vi "MakeMatlabParameterBundle.vi"(9 "value":variant, 10 "name":string, 11 "MatlabType":T2) -> (3 "MatlabDataBundle":T1)   [LabVIEW 2017]
uses:
  Types/MatlabDataType.ctl
  Types/MatlabDataBundle.ctl
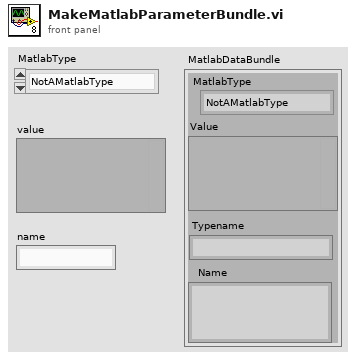
[diagram p1: front panel]
types:
  T1 = typedef "MatlabDataBundle.ctl" = cluster{"MatlabType":T2, "Value":variant, "Name":string, "Typename":string}
  T2 = typedef "MatlabDataType.ctl" = enum16{"NotAMatlabType", "Real", "Complex", "String", "Boolean"}
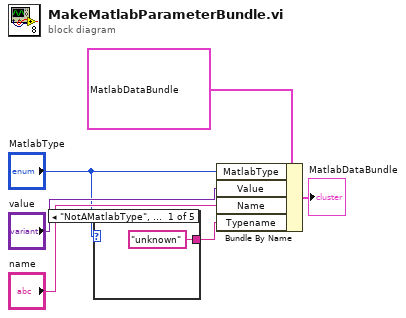
[diagram p0: block diagram]
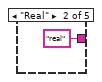
[diagram p2: hidden frame]
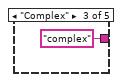
[diagram p3: hidden frame]
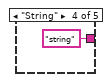
[diagram p4: hidden frame]
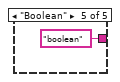
[diagram p5: hidden frame]
diagram:
  n1 = case shown="\"NotAMatlabType\", Default" "MatlabType" {
    tunnel: ["unknown" ("Typename") "real" ("Typename") "complex" ("Typename") "string" ("Typename") "boolean" ("Typename")] -> w1
    frame "NotAMatlabType", Default {
    }
    frame "Real" {
    }
    frame "Complex" {
    }
    frame "String" {
    }
    frame "Boolean" {
    }
  }
  n2 = Bundle By Name(cluster=T1 {"MatlabType"=enum."NotAMatlabType", "Value"=variant, "Name"="", "Typename"=""} ("input cluster"), "MatlabType"="MatlabType", "Value"="value", "Name"="name", "Typename"=w1) -> (→"MatlabDataBundle":T1)
